vi "speakerRecognition.vi"() -> ()   [LabVIEW 2020]
panel:
  out "record main password":bool
  in  "change password using audio":bool
  out "redy to record":bool
  in  "recording main password":bool
  in  "Radio Buttons":enum32{"reset password", "password", "OFF"}(radio)
  in  "stop":bool
  out "main voice":dbl[](graph)
  out "verified?":bool
  in  "record password":bool
  out "passowrd":dbl[](graph)
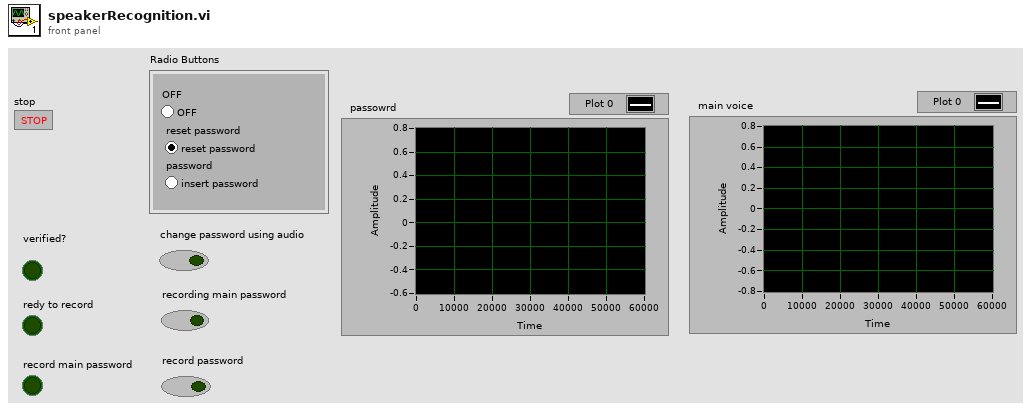
[diagram p1: front panel]
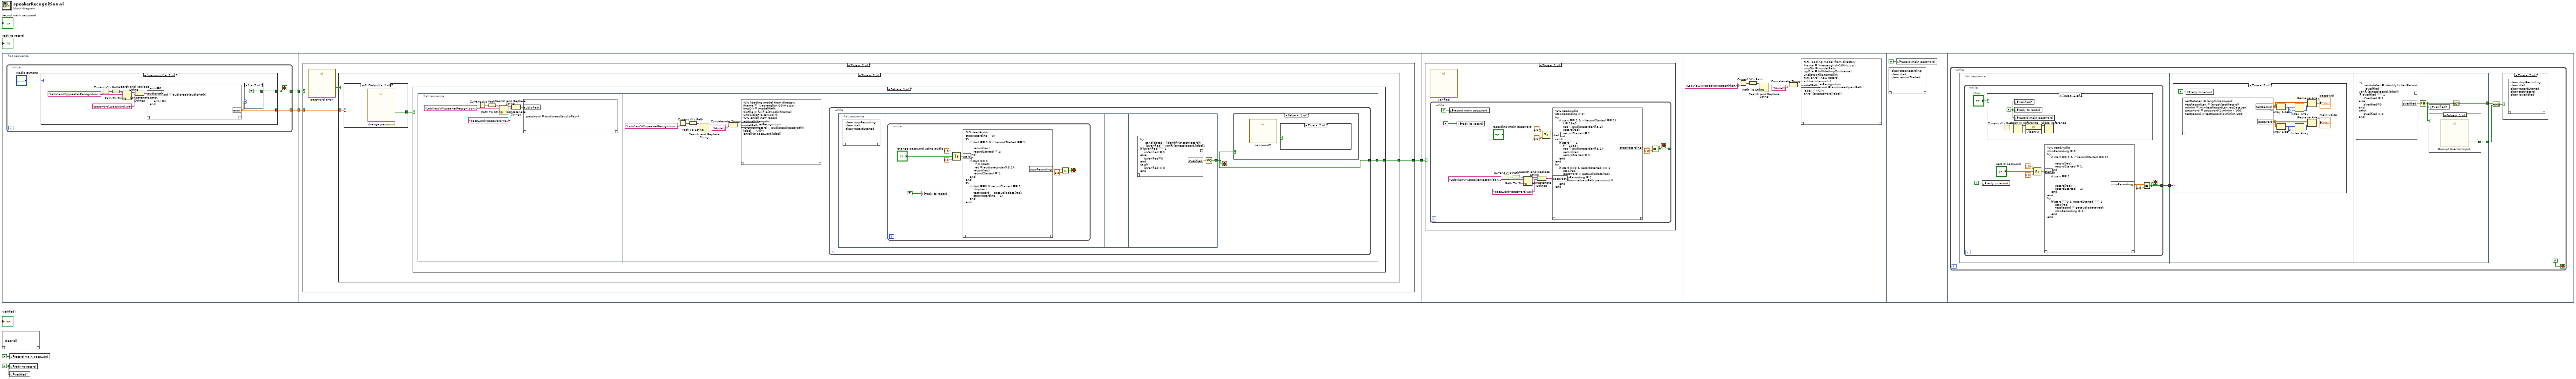
[diagram p0: block diagram]
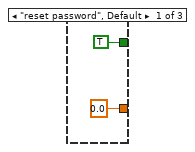
[diagram p2: hidden frame]
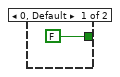
[diagram p3: hidden frame]
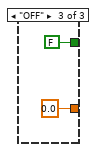
[diagram p4: hidden frame]
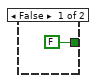
[diagram p5: hidden frame]
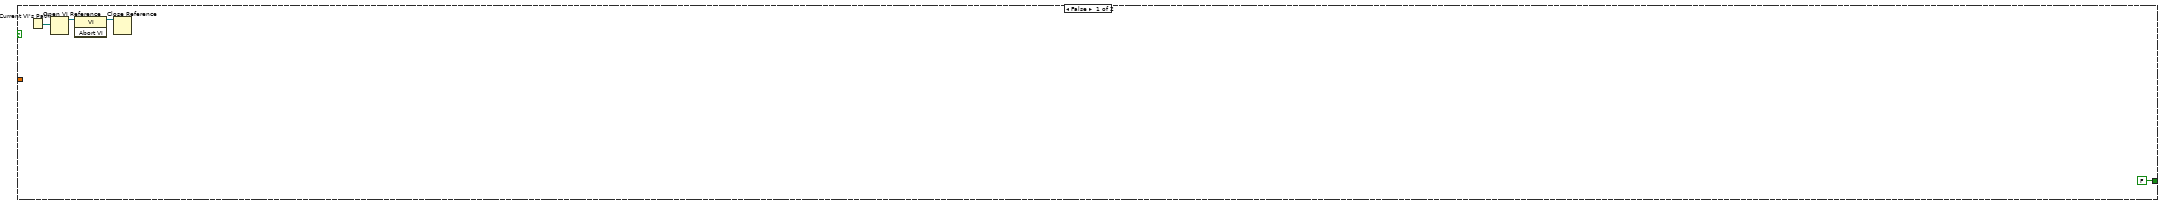
[diagram p6: hidden frame]
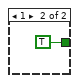
[diagram p7: hidden frame]
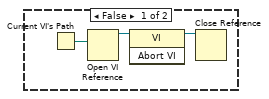
[diagram p8: hidden frame]
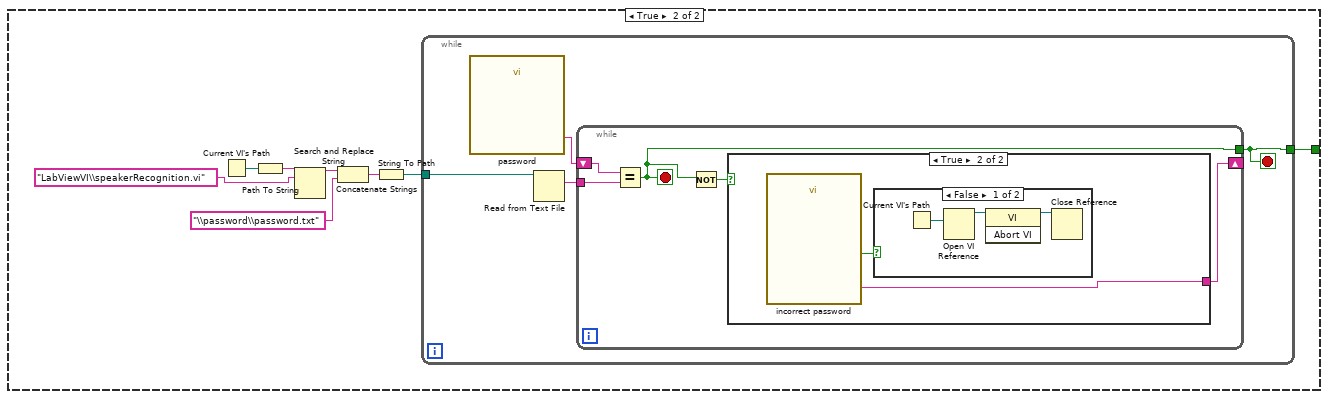
[diagram p10: hidden frame]
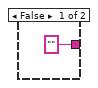
[diagram p11: hidden frame]
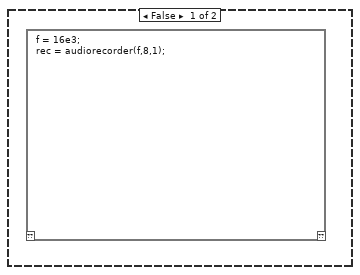
[diagram p13: hidden frame]
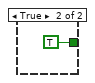
[diagram p17: hidden frame]
diagram:
  w2 = FALSE ("redy to record")
  n1 = flat-sequence {
    tunnel: [w7] -> w5
    tunnel: [w6] -> w3
    tunnel: w5 -> [w27]
    tunnel: [w26] -> w4
    tunnel: w3 -> [w25]
    tunnel: w4 -> [w93]
    frame #0 {
      n2 = while {
        tunnel: [w8] -> w7
        tunnel: [w9] -> w6
        stop <- w8 stop-if-true
        n3 = case shown="\"password\"" "Radio Buttons" {
          tunnel: [TRUE w20 FALSE] -> w8
          tunnel: [0.0 w19 0.0] -> w9
          frame "reset password", Default {
          }
          frame "password" {
            n4 = Current VI's Path() -> (path=w13:path)
            n5 = Path To String(path=w13) -> (string=w18:string)
            n6 = Search and Replace String(input string=w18, search string="LabViewVI\\speakerRecognition.vi" ("substring (\"\")")) -> (result string=w17:string)  [unwired: 6 in, 3 out]
            n7 = Concatenate Strings(w17, "password\\password.wav" ("string")) -> (w14:string)
            n8 = script code="error=0\ntry\n    password = audioread(audioPath)\ncatch \n    error =1\nend"("audioPath"=w14) -> ("error"=w19:dbl)  [unwired: 1 in, 1 out]
            n9 = case shown="1" w19 {
              tunnel: [FALSE TRUE] -> w20
              frame 0, Default {
              }
              frame 1 {
              }
            }
          }
          frame "OFF" {
          }
        }
      }
    }
    frame #1 {
      n10 = case shown="True" w27 {
        tunnel: [FALSE w30] -> w26
        tunnel: w25 -> [_ w29]
        frame False {
        }
        frame True {
          n11 = call "password error"() -> ("set password"=w31:bool)  [unwired: 18 in, 1 out]
          n12 = case shown="True" w31 {
            tunnel: [FALSE w38] -> w30
            tunnel: w29 -> [_ w36]
            frame False {
              n13 = Current VI's Path() -> (path=w35:path)
              n14 = Open VI Reference(vi path=w35) -> (vi reference=w34:refnum<vi>)  [unwired: 5 in, 1 out]
              n15 = invoke class="VI" method="Abort VI"(reference=w34) -> (reference out=w33:refnum<vi>)  [unwired: 2 in, 2 out]
              n16 = Close Reference(reference=w33) -> ()  [unwired: 1 in, 1 out]
            }
            frame True {
              n17 = case shown="0, Default" w36 {
                tunnel: [w39 TRUE ("Numeric")] -> w37
                frame 0, Default {
                  n18 = call "change password"() -> ("Numeric"=w39:bool)  [unwired: 18 in, 1 out]
                }
                frame 1 {
                }
              }
              n19 = case shown="False" w37 {
                tunnel: [w41 w70] -> w38
                frame False {
                  n20 = flat-sequence {
                    tunnel: [w54] -> w41
                    frame #0 {
                      n21 = Current VI's Path() -> (path=w42:path)
                      n22 = Path To String(path=w42) -> (string=w47:string)
                      n23 = Search and Replace String(input string=w47, search string="LabViewVI\\speakerRecognition.vi" ("substring (\"\")")) -> (result string=w46:string)  [unwired: 6 in, 3 out]
                      n24 = Concatenate Strings(w46, "password\\password.wav" ("string")) -> (w43:string)
                      n25 = script code="password = audioread(audioPath)"("audioPath"=w43) -> ()  [unwired: 1 in, 1 out]
                    }
                    frame #1 {
                      n26 = Current VI's Path() -> (path=w52:path)
                      n27 = Path To String(path=w52) -> (string=w50:string)
                      n28 = Search and Replace String(input string=w50, search string="LabViewVI\\speakerRecognition.vi" ("substring (\"\")")) -> (result string=w51:string)  [unwired: 6 in, 3 out]
                      n29 = Concatenate Strings(w51, "Model\\" ("string")) -> (w53:string)
                      n30 = script code="%% loading model from directory\nfname = 'ivec-english-16kHz.zip';\ntmpDir = modelPath;\nzipFile = fullfile(tmpDir,fname);\nunzip(zipFile,tempdir);\n%% enroll new record\naddpath(tempdir)\nsr = speakerRecognition;\n% enrollRecord = audioread(passPath);\nlabel = \"Ali\";\nenroll(sr,password,label)"("modelPath"=w53) -> ()  [unwired: 1 in, 1 out]
                    }
                    frame #2 {
                      n31 = while {
                        tunnel: [w55] -> w54
                        stop <- w55 stop-if-true
                        n32 = flat-sequence {
                          tunnel: [w68] -> w55
                          frame #0 {
                            n33 = script code="clear stopRecording\nclear start\nclear recordStarted"() -> ()  [unwired: 1 in, 1 out]
                          }
                          frame #1 {
                            n34 = while {
                              stop <- w62 stop-if-true
                              n35 = local write "redy to record"(TRUE ("record main password")) -> ()
                              n36 = Select(t=1.0, s="change password using audio", f=0.0) -> (s? t:f=w67:dbl)
                              n37 = script code="%% readAudio\nstopRecording = 0;\ntry\n    if start == 1 & ~(recordStarted == 1)\n\n        record(rec);\n        recordStarted = 1;\n    end\ncatch\n    if start == 1\n          f = 16e3;\n         rec = audiorecorder(f,8,1);\n        record(rec);\n        recordStarted = 1;\n    end\nend\ntry\n    if start ==0 & recordStarted == 1\n        stop(rec)\n        testRecord = getaudiodata(rec);\n        stopRecording = 1;\n    end\nend"("start"=w67) -> ("stopRecording"=w64:dbl)  [unwired: 1 in, 1 out]
                              n38 = Equal?(x=w64, y=1.0) -> (x = y?=w62:bool)
                            }
                          }
                          frame #2 {
                          }
                          frame #3 {
                            n39 = script code="try\n     candidates = identify(sr,testRecord);\n      isVerified = verify(sr,testRecord,label);\nif isVerified == 1\n    isVerified = 1\nelse\n    isVerified=0\nend\ncatch\n    isVerified = 0\nend"() -> ("isVerified"=w69:dbl)  [unwired: 1 in, 1 out]
                            n40 = Not Equal To 0?(x=w69) -> (x != 0?=w68:bool)
                          }
                        }
                        n41 = case shown="False" w55 {
                          frame False {
                            n42 = call "password2"() -> ("Retry"=w56:bool)  [unwired: 18 in, 1 out]
                            n43 = case shown="True" w56 {
                              frame False {
                                n44 = Current VI's Path() -> (path=w59:path)
                                n45 = Open VI Reference(vi path=w59) -> (vi reference=w58:refnum<vi>)  [unwired: 5 in, 1 out]
                                n46 = invoke class="VI" method="Abort VI"(reference=w58) -> (reference out=w57:refnum<vi>)  [unwired: 2 in, 2 out]
                                n47 = Close Reference(reference=w57) -> ()  [unwired: 1 in, 1 out]
                              }
                              frame True {
                              }
                            }
                          }
                          frame True {
                          }
                        }
                      }
                    }
                  }
                }
                frame True {
                  n48 = Current VI's Path() -> (path=w77:path)
                  n49 = Path To String(path=w77) -> (string=w75:string)
                  n50 = Search and Replace String(input string=w75, search string="LabViewVI\\speakerRecognition.vi" ("substring (\"\")")) -> (result string=w74:string)  [unwired: 6 in, 3 out]
                  n51 = Concatenate Strings(w74, "\\password\\password.txt" ("string")) -> (w76:string)
                  n52 = String To Path(string=w76) -> (path=w71:path)
                  n53 = while {
                    tunnel: w71 -> [w79]
                    tunnel: [w78] -> w70
                    stop <- w78 stop-if-true
                    n54 = call "password"() -> ("password"=w80:string)  [unwired: 17 in, 2 out]
                    n55 = Read from Text File(file (use dialog)=w79) -> (text=w81:string)  [unwired: 3 in, 3 out]
                    n56 = while {
                      tunnel: w81 -> [w86]
                      shift-right: [w84] -> _
                      shift-left: w80 -> [w85]
                      tunnel: [w82] -> w78
                      stop <- w82 stop-if-true
                      n57 = Equal?(x=w85, y=w86) -> (x = y?=w82:bool)
                      n58 = Not(x=w82) -> (.not. x?=w83:bool)
                      n59 = case shown="True" w83 {
                        tunnel: ["" ("password") w88] -> w84
                        frame False {
                        }
                        frame True {
                          n60 = call "incorrect password"() -> ("password"=w88:string, "OK"=w89:bool)  [unwired: 17 in, 1 out]
                          n61 = case shown="False" w89 {
                            frame False {
                              n62 = Current VI's Path() -> (path=w92:path)
                              n63 = Open VI Reference(vi path=w92) -> (vi reference=w91:refnum<vi>)  [unwired: 5 in, 1 out]
                              n64 = invoke class="VI" method="Abort VI"(reference=w91) -> (reference out=w90:refnum<vi>)  [unwired: 2 in, 2 out]
                              n65 = Close Reference(reference=w90) -> ()  [unwired: 1 in, 1 out]
                            }
                            frame True {
                            }
                          }
                        }
                      }
                    }
                  }
                }
              }
            }
          }
        }
      }
    }
    frame #2 {
      n66 = case shown="True" w93 {
        frame False {
          n67 = script code="f = 16e3;\nrec = audiorecorder(f,8,1);"() -> ()  [unwired: 1 in, 1 out]
        }
        frame True {
          n68 = call "verified"() -> ()  [unwired: 18 in, 2 out]
          n69 = while {
            tunnel: [w103] -> _
            stop <- w103 stop-if-true
            n70 = local write "record main password"(TRUE ("record main password")) -> ()
            n71 = local write "redy to record"(FALSE ("record main password")) -> ()
            n72 = Current VI's Path() -> (path=w96:path)
            n73 = Path To String(path=w96) -> (string=w100:string)
            n74 = Search and Replace String(input string=w100, search string="LabViewVI\\speakerRecognition.vi" ("substring (\"\")")) -> (result string=w99:string)  [unwired: 6 in, 3 out]
            n75 = Concatenate Strings(w99, "password\\password.wav" ("string")) -> (w95:string)
            n76 = Select(t=1.0, s="recording main password", f=0.0) -> (s? t:f=w108:dbl)
            n77 = script code="%% readAudio\nstopRecording = 0;\ntry\n    if start == 1 & ~(recordStarted == 1)\n        f = 16e3;\n        rec = audiorecorder(f,8,1);\n        record(rec);\n        recordStarted = 1;\n    end\ncatch\n    if start == 1\n        f = 16e3;\n        rec = audiorecorder(f,8,1);\n        record(rec);\n        recordStarted = 1;\n    end\nend\ntry\n    if start ==0 & recordStarted == 1\n        stop(rec)\n        password = getaudiodata(rec);\n        stopRecording = 1;\n        audiowrite(passPath,password,f)\n    end\nend"("start"=w108, "passPath"=w95) -> ("stopRecording"=w105:dbl)  [unwired: 1 in, 1 out]
            n78 = Equal?(x=w105, y=1.0) -> (x = y?=w103:bool)
          }
        }
      }
    }
    frame #3 {
      n79 = Current VI's Path() -> (path=w110:path)
      n80 = Path To String(path=w110) -> (string=w114:string)
      n81 = Search and Replace String(input string=w114, search string="LabViewVI\\speakerRecognition.vi" ("substring (\"\")")) -> (result string=w113:string)  [unwired: 6 in, 3 out]
      n82 = Concatenate Strings(w113, "Model\\" ("string")) -> (w109:string)
      n83 = script code="%% loading model from directory\nfname = 'ivec-english-16kHz.zip';\ntmpDir = modelPath;\nzipFile = fullfile(tmpDir,fname);\nunzip(zipFile,tempdir);\n%% enroll new record\naddpath(tempdir)\nsr = speakerRecognition;\n% enrollRecord = audioread(passPath);\nlabel = \"Ali\";\nenroll(sr,password,label)"("modelPath"=w109) -> ()  [unwired: 1 in, 1 out]
    }
    frame #4 {
      n84 = script code="clear stopRecording\nclear start\nclear recordStarted"() -> ()  [unwired: 1 in, 1 out]
      n85 = local write "record main password"(FALSE ("record main password")) -> ()
    }
    frame #5 {
      n86 = while {
        stop <- FALSE stop-if-true
        n87 = flat-sequence {
          tunnel: [w121] -> w117
          tunnel: w117 -> [w135]
          tunnel: [w149] -> w120
          tunnel: [w150] -> w119
          frame #0 {
            n88 = while {
              tunnel: [w123] -> w121
              stop <- w123 stop-if-true
              n89 = local write "redy to record"(TRUE ("redy to record")) -> ()
              n90 = case shown="True" "stop" {
                frame False {
                }
                frame True {
                  w131 = FALSE ("redy to record")
                  n91 = Current VI's Path() -> (path=w134:path)
                  n92 = Open VI Reference(vi path=w134) -> (vi reference=w133:refnum<vi>)  [unwired: 5 in, 1 out]
                  n93 = local write "verified?"(w131) -> ()
                  n94 = local write "redy to record"(w131) -> ()
                  n95 = local write "record main password"(w131) -> ()
                  n96 = invoke class="VI" method="Abort VI"(reference=w133) -> (reference out=w132:refnum<vi>)  [unwired: 2 in, 2 out]
                  n97 = Close Reference(reference=w132) -> ()  [unwired: 1 in, 1 out]
                }
              }
              n98 = Select(t=1.0, s="record password", f=0.0) -> (s? t:f=w130:dbl)
              n99 = script code="%% readAudio\nstopRecording = 0;\ntry\n    if start == 1 & ~(recordStarted == 1)\n\n        record(rec);\n        recordStarted = 1;\n    end\ncatch\n    if start == 1\n\n\n        record(rec);\n        recordStarted = 1;\n    end\nend\ntry\n    if start ==0 & recordStarted == 1\n        stop(rec)\n        testRecord = getaudiodata(rec);\n        stopRecording = 1;\n    end\nend"("start"=w130) -> ("stopRecording"=w127:dbl)  [unwired: 1 in, 1 out]
              n100 = Equal?(x=w127, y=1.0) -> (x = y?=w123:bool)
            }
          }
          frame #1 {
            n101 = case shown="True" w135 {
              frame False {
              }
              frame True {
                n102 = script code="recDataLen = length(password)\ntestRecordLen = length(testRecord)\nminim = min(testRecordLen,recDataLen)\npassword = password(1:minim - 100)\ntestRecord = testRecord(1:minim-100)"() -> ("testRecord"=w146:dbl[][], "password"=w140:dbl[][])  [unwired: 1 in, 1 out]
                n103 = local write "redy to record"(FALSE ("redy to record")) -> ()
                n104 = Array Size(array=w146) -> (size(s)=w145:i32[])
                n105 = Array Size(array=w140) -> (size(s)=w139:i32[])
                n106 = Index Array(array=w145, index=0) -> (element=w143:i32)
                n107 = Index Array(array=w139, index=0) -> (element=w138:i32)
                n108 = Reshape Array(w146, w143) -> (→"passowrd":dbl[])
                n109 = Reshape Array(w140, w138) -> (→"main voice":dbl[])
              }
            }
          }
          frame #2 {
            n110 = script code="try\n     candidates = identify(sr,testRecord);\n      isVerified = verify(sr,testRecord,label);\nif isVerified == 1\n    isVerified = 1\nelse\n    isVerified=0\nend\ncatch\n    isVerified = 0\nend"() -> ("isVerified"=w148:dbl)  [unwired: 1 in, 1 out]
            n111 = Not Equal To 0?(x=w148) -> (x != 0?=w147:bool)
            n112 = local write "verified?"(w147) -> ()
            n113 = case shown="False" w147 {
              tunnel: [w151 TRUE ("Clacle")] -> w150
              frame False {
                n114 = call "Prompt User for Input"() -> ("OK"=w151:bool)  [unwired: 18 in, 1 out]
              }
              frame True {
              }
            }
            n115 = Not(x=w147) -> (.not. x?=w149:bool)
          }
        }
        n116 = And(x=w120, y=w119) -> (x .and. y?=w118:bool)
        n117 = case shown="True" w118 {
          frame False {
          }
          frame True {
            n118 = script code="clear stopRecording\nclear start\nclear recordStarted\nclear testRecord\nclear isVeridied"() -> ()  [unwired: 1 in, 1 out]
          }
        }
      }
    }
  }
  n119 = script code="clear all"() -> ()  [unwired: 1 in, 1 out]
  n120 = local write "record main password"(FALSE ("record main password")) -> ()
  n121 = local write "redy to record"(w2) -> ()
  n122 = local write "verified?"(w2) -> ()
